vi "Write Buffer.vi"(8 "error in (no error)":errorcluster, 10 "Buffer":u8[](array[numeric]) format="%x", 11 "CIFfifo in":refnum<class "CIFfifo.lvclass">) -> (0 "error out":errorcluster, 3 "CIFfifo out":refnum<class "CIFfifo.lvclass">)   [LabVIEW 2021, in "CIFfifo.lvclass"]
uses:
  CIFfifo.lvclass
  CIFfifo.lvclass/CIFfifo.ctl
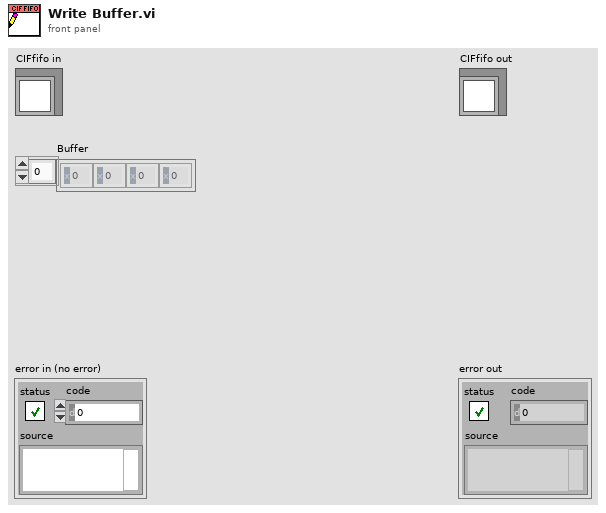
[diagram p1: front panel]
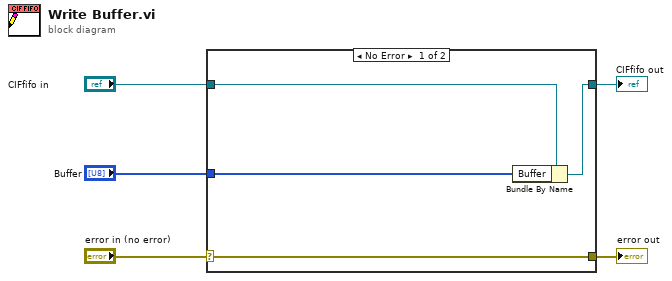
[diagram p0: block diagram]
diagram:
  n1 = case shown="No Error" "error in (no error)" {
    selector: "error in (no error)" -> [w9 w10]
    tunnel: [w9 w10] -> w4
    tunnel: [w7 w11] -> w2
    tunnel: "CIFfifo in" -> [w8 w11]
    tunnel: "Buffer" -> [w6 _]
    frame No Error {
      n2 = Bundle By Name(cluster=w8, "Buffer"=w6) -> (w7:refnum<class "CIFfifo.lvclass">)
    }
    frame Error {
    }
  }
  "error out" <- w4
  "CIFfifo out" <- w2
